vi "SSL Detection Frame.vi"(8 "error in":errorcluster, 9 "Array":u8[](array[numeric]) format="%02x") -> (0 "error out":errorcluster, 3 "Detection Frame":T1)   [LabVIEW 2016]
uses:
  SSL Detection Frame.ctl
  SSL Detection Robot.ctl
  SSL Detection Ball.ctl
  Varint Decoder uint32.vi
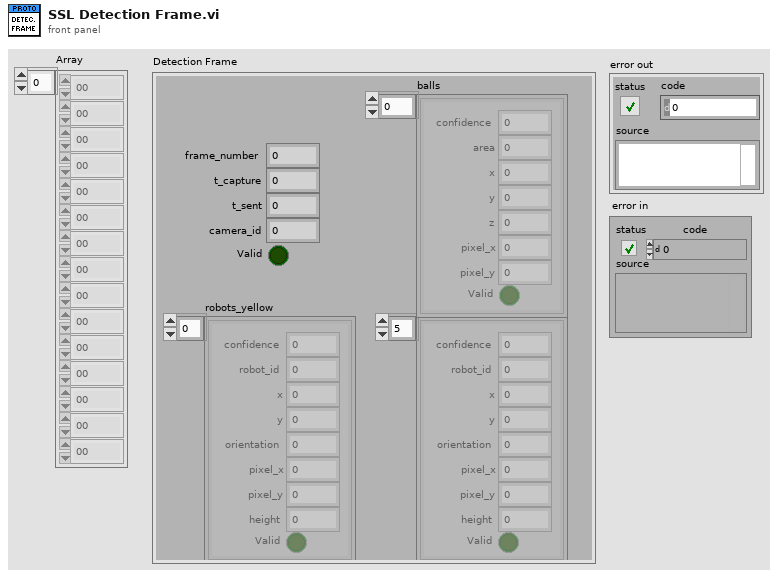
[diagram p1: front panel]
types:
  T1 = typedef "SSL Detection Frame.ctl" = cluster{"frame_number":u32, "t_capture":dbl, "t_sent":dbl, "camera_id":u32, "robots_yellow":T2[], "robots_blue":T2[], "balls":T3[], "Valid":bool}
  T2 = typedef "SSL Detection Robot.ctl" = cluster{"x":dbl, "robot_id":u32, "confidence":sgl, "y":sgl, "orientation":sgl, "pixel_x":sgl, "pixel_y":sgl, "height":sgl, "Valid":bool}
  T3 = typedef "SSL Detection Ball.ctl" = cluster{"x":sgl, "area":u32, "confidence":sgl, "y":sgl, "z":sgl, "pixel_x":sgl, "pixel_y":sgl, "Valid":bool}
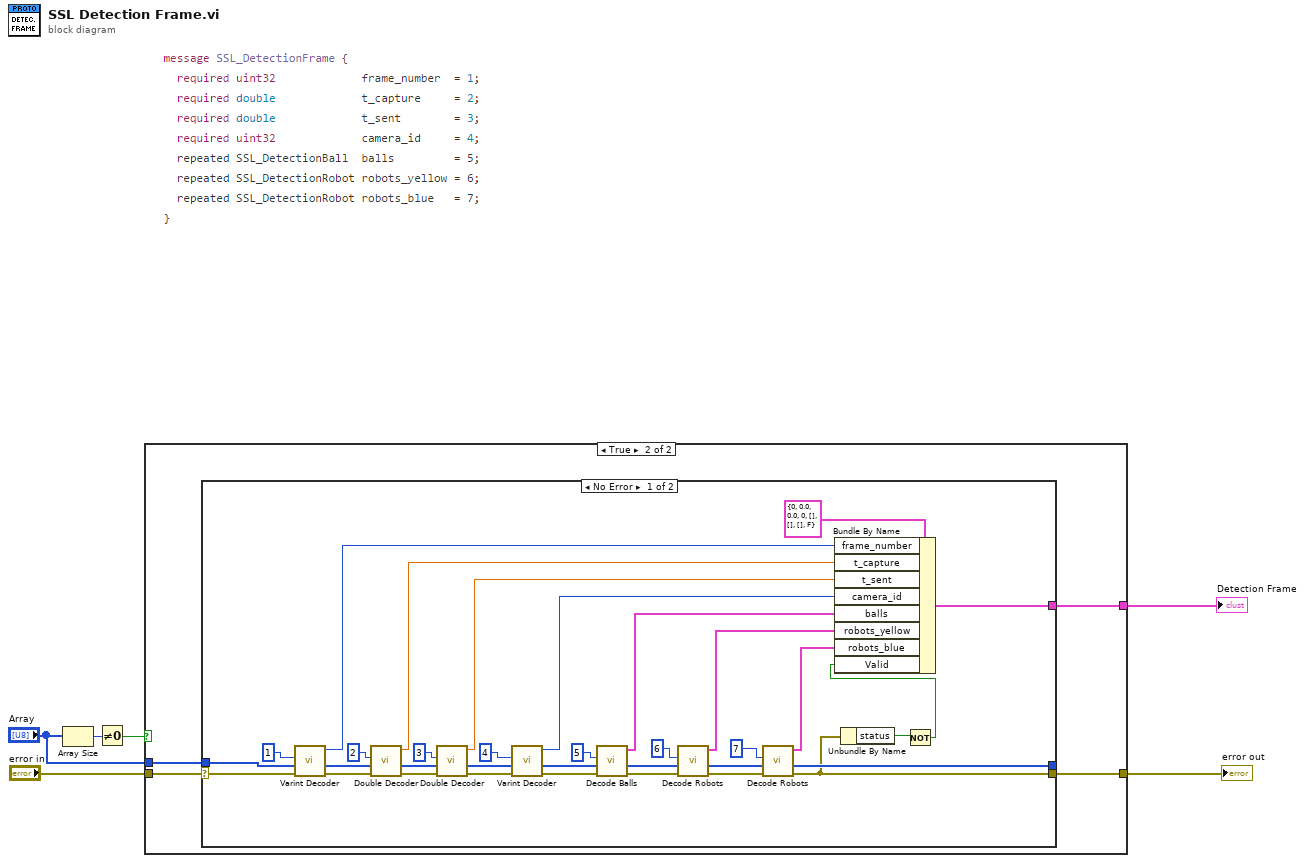
[diagram p0: block diagram]
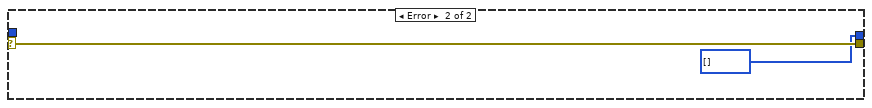
[diagram p3: hidden frame]
diagram:
  n1 = Array Size(array="Array") -> (size(s)=w4:i32)
  n2 = Not Equal To 0?(x=w4) -> (x != 0?=w2:bool)
  n3 = case shown="True" w2 {
    tunnel: "error in" -> [_ w10]
    tunnel: "Array" -> [_ w9]
    tunnel: [_ w8] -> w3
    tunnel: [_ w7] -> w1
    frame False {
    }
    frame True {
      n4 = case shown="No Error" w10 {
        selector: w10 -> [w43 w46]
        tunnel: [w14 w46] -> w8
        tunnel: [w16 u8[] [] ("array w/ subset deleted")] -> _
        tunnel: w9 -> [w15 _]
        tunnel: [w11 _] -> w7
        frame No Error {
          n5 = call-poly "Varint Decoder.vi"("error in (no error)"=w43, "Array"=w15, "Key"=1) -> ("error out"=w42:errorcluster, "array w/ subset deleted"=w26:u8[], "Varint"=w31:u32)  [unwired: 5 in, 1 out]
          n6 = call "Double Decoder.vi"("error in (no error)"=w42, "Array"=w26, "Key"=2) -> ("error out"=w41:errorcluster, "array w/ subset deleted"=w27:u8[], "Double"=w32:dbl)  [unwired: 5 in, 1 out]
          n7 = call "Double Decoder.vi"("error in (no error)"=w41, "Array"=w27, "Key"=3) -> ("error out"=w40:errorcluster, "array w/ subset deleted"=w28:u8[], "Double"=w33:dbl)  [unwired: 5 in, 1 out]
          n8 = call-poly "Varint Decoder.vi"("error in (no error)"=w40, "Array"=w28, "Key"=4) -> ("error out"=w36:errorcluster, "array w/ subset deleted"=w29:u8[], "Varint"=w34:u32)  [unwired: 5 in, 1 out]
          n9 = call "Decode Balls.vi"("error in"=w36, "array"=w29, "Key"=5) -> ("error out"=w24:errorcluster, "array w/ subset deleted out"=w23:u8[], "Array"=w30:T3[])  [unwired: 6 in]
          n10 = call "Decode Robots.vi"("error in"=w24, "array"=w23, "Key"=6) -> ("error out"=w21:errorcluster, "array w/ subset deleted out"=w20:u8[], "Robots"=w18:T2[])  [unwired: 6 in]
          n11 = call "Decode Robots.vi"("error in"=w21, "array"=w20, "Key"=7) -> ("error out"=w14:errorcluster, "array w/ subset deleted out"=w16:u8[], "Robots"=w17:T2[])  [unwired: 6 in]
          n12 = Unbundle By Name(w14) -> ("status"=w13:bool)
          n13 = Not(x=w13) -> (.not. x?=w12:bool)
          n14 = Bundle By Name(cluster=T1 {"frame_number"=0, "t_capture"=0.0, "t_sent"=0.0, "camera_id"=0, "robots_yellow"=[], "robots_blue"=[], "balls"=[], "Valid"=FALSE} ("Detection Frame 2"), "frame_number"=w31, "t_capture"=w32, "t_sent"=w33, "camera_id"=w34, "balls"=w30, "robots_yellow"=w18, "robots_blue"=w17, "Valid"=w12) -> (w11:T1)
        }
        frame Error {
        }
      }
    }
  }
  "error out" <- w3
  "Detection Frame" <- w1
